vi "UpdateLinkCameraStatus.vi"(8 "error in (no error)":errorcluster, 10 "LinkCameraStatus":T1=enum."Connected", 11 "ICameraTestingUI in":refnum<class "ICameraTestingUI.lvclass">) -> (0 "error out":errorcluster, 3 "ICameraTestingUI out":refnum<class "ICameraTestingUI.lvclass">)   [LabVIEW 2020, in "ICameraTestingUI.lvlib" / "ICameraTestingUI.lvclass"]
uses:
  ICameraTestingUI.lvclass
  TypeDef/LinkCameraStatus.ctl
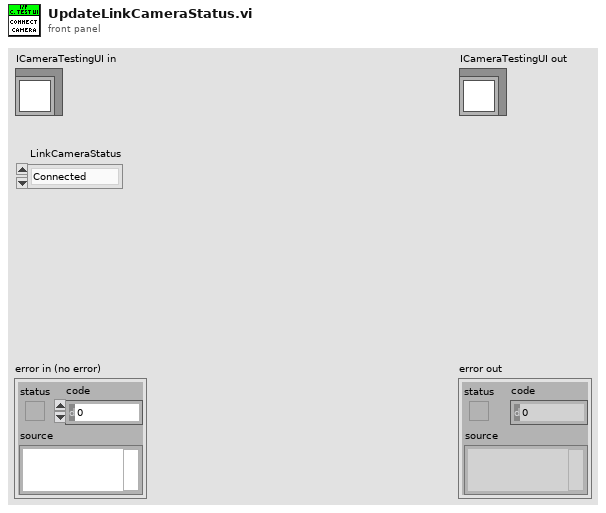
[diagram p1: front panel]
types:
  T1 = typedef "ICameraTestingUI.lvlib/ICameraTestingUI.lvclass/LinkCameraStatus.ctl" = enum8{"Disconnected", "Connected", "Error"}
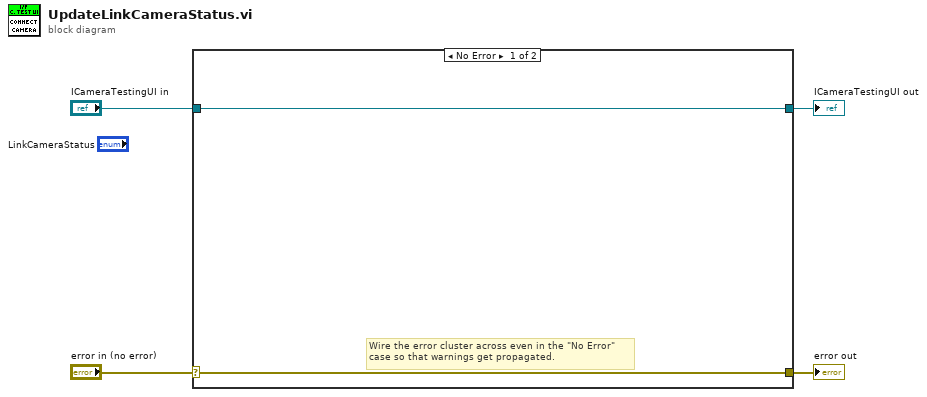
[diagram p0: block diagram]
diagram:
  n1 = case shown="No Error" "error in (no error)" {
    selector: "error in (no error)" -> [w5 w8]
    tunnel: [w5 w8] -> w3
    tunnel: [w6 w7] -> w1
    tunnel: "ICameraTestingUI in" -> [w6 w7]
    frame No Error {
      # "Wire the error cluster across even in the \"No Error\"\ncase so that warnings get propagated."
    }
    frame Error {
    }
  }
  "error out" <- w3
  "ICameraTestingUI out" <- w1
